vi "湿度显示前面板.vi"(0 "通道设置":u8=1 min=1 max=100, 1 "通讯设置":T1={"COM1", "Baud Rate"=19200, "Slave Address"=255}) -> (3 "光谱图像":cluster{dbl[], u16[]}(graph))   [LabVIEW 2018]
uses:
  <vilib>/Utility/file.llb/Read Delimited Spreadsheet (DBL).vi
  <vilib>/Utility/file.llb/Write To Spreadsheet File (DBL).vi
panel:
  in  "阈值":u16
  in  "连接":bool
  in  "选项卡控件":T2(tab)
  out "3通道":dbl[](array[numeric]) format="%#_7g"
  out "2通道":dbl[](array[numeric]) format="%#_7g"
  out "1通道":dbl[](array[numeric])=[1546.786, 1549.013] format="%#_7g"
  out "4通道":dbl[](array[numeric]) format="%#_7g"
  out "波形图表 20":dbl(graph)
  out "波形图表 19":dbl(graph)
  out "波形图表 18":dbl(graph)
  out "波形图表 17":dbl(graph)
  out "波形图表 16":dbl(graph)
  out "波形图表 15":dbl(graph)
  out "波形图表 14":dbl(graph)
  out "波形图表 13":dbl(graph)
  out "波形图表 12":dbl(graph)
  out "波形图表 11":dbl(graph)
  out "波形图表 10":dbl(graph)
  out "波形图表 9":dbl(graph)
  out "波形图表 8":dbl(graph)
  out "波形图表 7":dbl(graph)
  out "波形图表 6":dbl(graph)
  out "波形图表 5":dbl(graph)
  out "湿度1":dbl
  out "温度1":dbl
  out "湿度2":dbl
  out "温度2":dbl
  out "湿度3":dbl
  out "温度3":dbl
  out "湿度4":dbl
  out "温度4":dbl
  out "湿度5":dbl
  out "温度5":dbl
  out "湿度6":dbl
  out "温度6":dbl
  out "湿度7":dbl
  out "温度7":dbl
  out "湿度8":dbl
  out "温度8":dbl
  out "湿度9":dbl
  out "温度9":dbl
  out "湿度10":dbl
  out "温度10":dbl
  out "波形图表 2":dbl(graph)
  out "波形图表 3":dbl(graph)
  out "波形图表 4":dbl(graph)
  out "波形图表":dbl(graph)
  out "波形图表 40":dbl(graph)
  out "波形图表 39":dbl(graph)
  out "波形图表 38":dbl(graph)
  out "波形图表 37":dbl(graph)
  out "波形图表 36":dbl(graph)
  out "波形图表 35":dbl(graph)
  out "波形图表 34":dbl(graph)
  out "波形图表 33":dbl(graph)
  out "波形图表 32":dbl(graph)
  out "波形图表 31":dbl(graph)
  out "波形图表 30":dbl(graph)
  out "波形图表 29":dbl(graph)
  out "波形图表 28":dbl(graph)
  out "波形图表 27":dbl(graph)
  out "波形图表 26":dbl(graph)
  out "波形图表 25":dbl(graph)
  out "波形图表 24":dbl(graph)
  out "波形图表 23":dbl(graph)
  out "波形图表 22":dbl(graph)
  out "波形图表 21":dbl(graph)
  out "湿度5 2":dbl
  out "温度5 2":dbl
  out "湿度6 2":dbl
  out "温度6 2":dbl
  out "湿度7 2":dbl
  out "温度7 2":dbl
  out "湿度8 2":dbl
  out "温度8 2":dbl
  out "湿度9 2":dbl
  out "温度9 2":dbl
  out "湿度10 2":dbl
  out "温度10 2":dbl
  out "湿度1 2":dbl
  out "温度1 2":dbl
  out "湿度2 2":dbl
  out "温度2 2":dbl
  out "湿度3 2":dbl
  out "温度3 2":dbl
  out "湿度4 2":dbl
  out "温度4 2":dbl
  out "波形图表 60":dbl(graph)
  out "波形图表 59":dbl(graph)
  out "波形图表 58":dbl(graph)
  out "波形图表 57":dbl(graph)
  out "波形图表 56":dbl(graph)
  out "波形图表 55":dbl(graph)
  out "波形图表 54":dbl(graph)
  out "波形图表 53":dbl(graph)
  out "波形图表 52":dbl(graph)
  out "波形图表 51":dbl(graph)
  out "波形图表 50":dbl(graph)
  out "波形图表 49":dbl(graph)
  out "波形图表 48":dbl(graph)
  out "波形图表 47":dbl(graph)
  out "波形图表 46":dbl(graph)
  out "波形图表 45":dbl(graph)
  out "波形图表 44":dbl(graph)
  out "波形图表 43":dbl(graph)
  out "波形图表 42":dbl(graph)
  out "波形图表 41":dbl(graph)
  out "温度1 3":dbl
  out "湿度1 3":dbl
  out "温度4 3":dbl
  out "湿度4 3":dbl
  out "温度3 3":dbl
  out "湿度3 3":dbl
  out "温度2 3":dbl
  out "湿度2 3":dbl
  out "湿度5 3":dbl
  out "温度5 3":dbl
  out "湿度6 3":dbl
  out "温度6 3":dbl
  out "湿度7 3":dbl
  out "温度7 3":dbl
  out "湿度8 3":dbl
  out "温度8 3":dbl
  out "湿度9 3":dbl
  out "温度9 3":dbl
  out "湿度10 3":dbl
  out "温度10 3":dbl
  out "波形图表 80":dbl(graph)
  out "波形图表 79":dbl(graph)
  out "波形图表 78":dbl(graph)
  out "波形图表 77":dbl(graph)
  out "波形图表 76":dbl(graph)
  out "波形图表 75":dbl(graph)
  out "波形图表 74":dbl(graph)
  out "波形图表 73":dbl(graph)
  out "波形图表 72":dbl(graph)
  out "波形图表 71":dbl(graph)
  out "波形图表 70":dbl(graph)
  out "波形图表 69":dbl(graph)
  out "波形图表 68":dbl(graph)
  out "波形图表 67":dbl(graph)
  out "波形图表 66":dbl(graph)
  out "波形图表 65":dbl(graph)
  out "波形图表 64":dbl(graph)
  out "波形图表 63":dbl(graph)
  out "波形图表 62":dbl(graph)
  out "波形图表 61":dbl(graph)
  out "温度1 4":dbl
  out "湿度1 4":dbl
  out "湿度2 4":dbl
  out "温度2 4":dbl
  out "湿度3 4":dbl
  out "温度3 4":dbl
  out "湿度4 4":dbl
  out "温度4 4":dbl
  out "湿度5 4":dbl
  out "温度5 4":dbl
  out "湿度6 4":dbl
  out "温度6 4":dbl
  out "湿度7 4":dbl
  out "温度7 4":dbl
  out "湿度8 4":dbl
  out "温度8 4":dbl
  out "湿度9 4":dbl
  out "温度9 4":dbl
  out "湿度10 4":dbl
  out "温度10 4":dbl
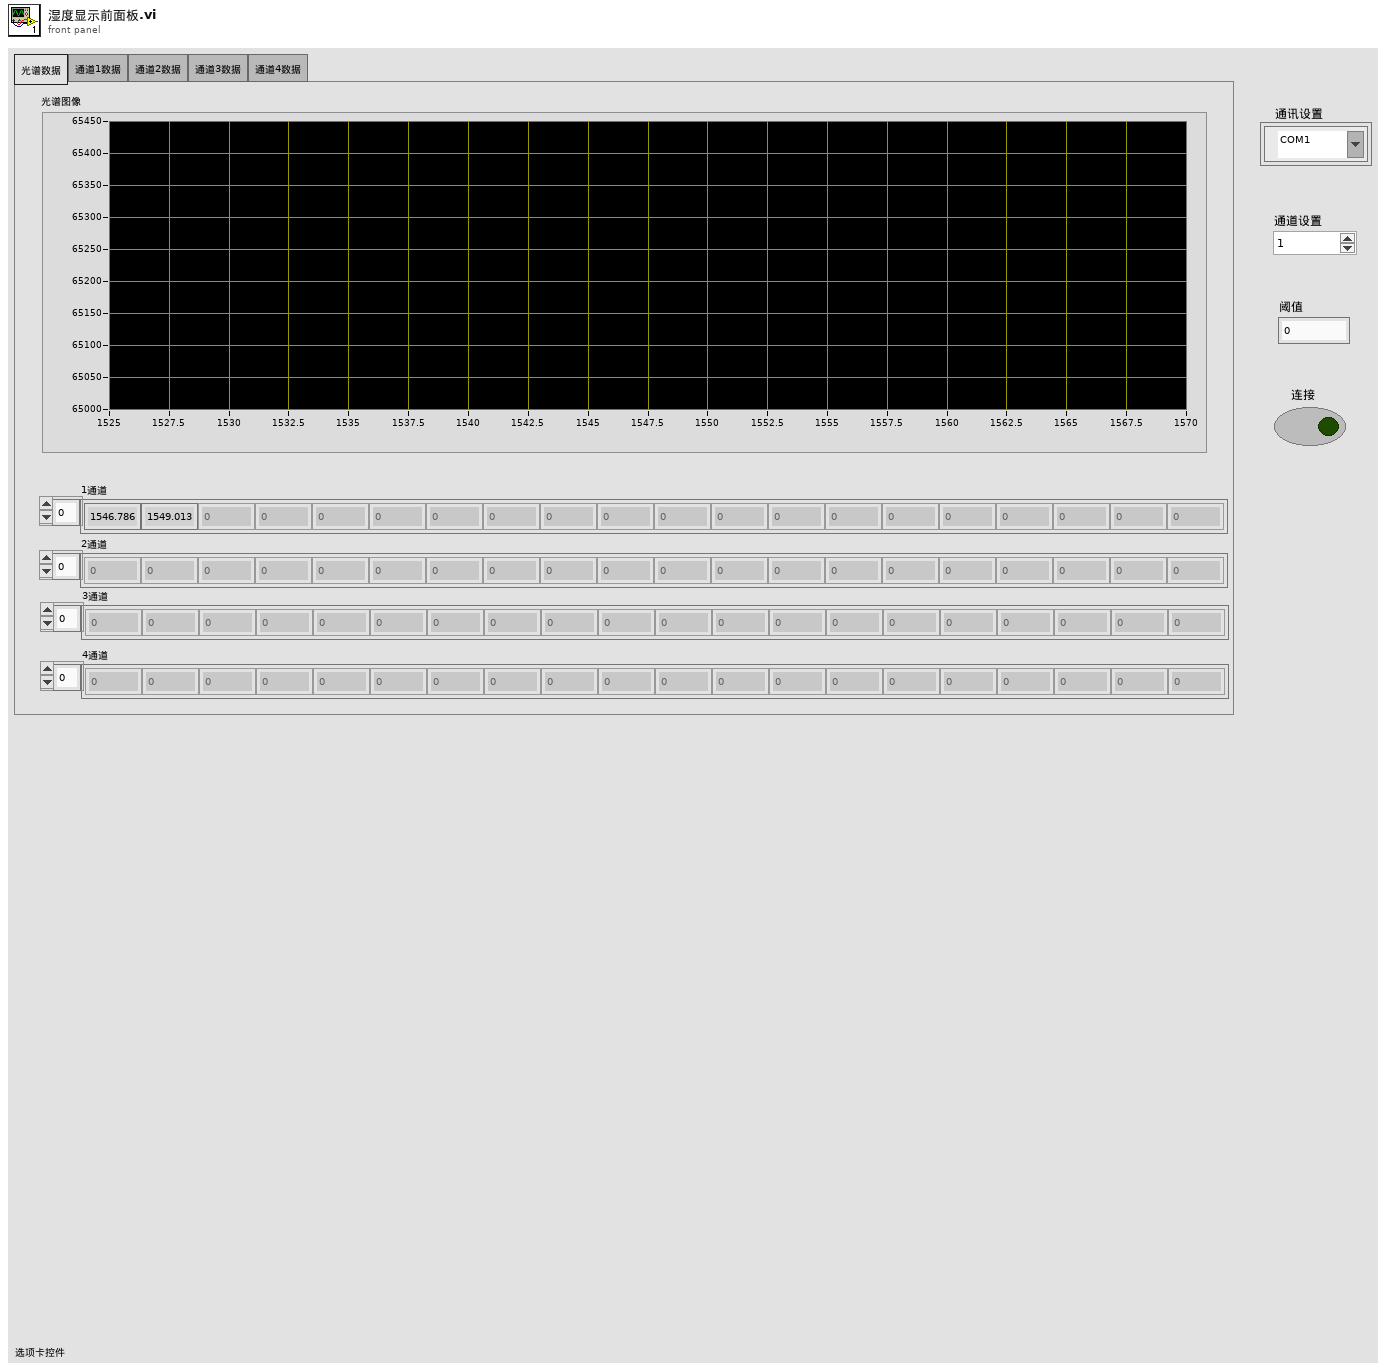
[diagram p1: front panel]
types:
  T1 = cluster{refnum<visa-resource-name>, "Baud Rate":u32, "Slave Address":u8}
  T2 = enum32{"光谱数据", "通道1数据", "通道2数据", "通道3数据", "通道4数据"}
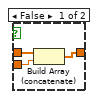
[diagram p2: hidden frame]
diagram:
  n1 = Unbundle By Name("通讯设置") -> ("Slave Address"=w5:u8)
  n2 = while {
    tunnel: w5 -> [w674]
    tunnel: "通讯设置" -> [w673]
    tunnel: [w672] -> w2
    tunnel: [w671] -> w1
    stop <- "连接" continue-if-true
    w678 = path "E:/湿度/四通道湿度结果" ("基路径")
    n3 = call "U8toHEX.vi"("data"=w674) -> ("HEX"=w726:string)  [unwired: 10 in]
    n4 = Concatenate Strings(w726, "B" ("write buffer")) -> (w736:string)
    n5 = call "CRC16.vi"("DATA"=w736) -> ("CRC-16"=w729:string)  [unwired: 1 in, 1 out]
    n6 = Concatenate Strings(w736, w729) -> (w732:string)
    n7 = call "Initialize.vi"("通讯设置 in"=w673) -> ("error out"=w734:errorcluster, "VISA resource name out"=w733:refnum<visa-resource-name>)  [unwired: 1 in, 3 out]
    n8 = VISA Write(VISA resource name=w733, write buffer=w732, error in (no error)=w734) -> (VISA resource name out=w730:refnum<visa-resource-name>, error out=w731:errorcluster)  [unwired: 1 out]
    n9 = flat-sequence {
      tunnel: w731 -> [w1062]
      tunnel: w730 -> [w1063]
      tunnel: [w1063] -> w744
      tunnel: [w1062] -> w743
      tunnel: [w1069] -> w728
      tunnel: [w1068] -> w727
      tunnel: [w1067] -> w725
      tunnel: w744 -> [w1066]
      tunnel: w743 -> [w1070]
      frame #0 {
        n10 = Wait (ms)(milliseconds to wait=u32 1000) -> ()  [unwired: 1 out]
      }
      frame #1 {
        n11 = property class="Instr" props=["Bytes at Port"](reference=w1066) -> (reference out=w1065:refnum<visa-resource-name>)  [unwired: 1 in, 2 out]
        n12 = VISA Read(VISA resource name=w1065, byte count=u32 8 ("Serial Settings:Number of Bytes at Serial Port"), error in (no error)=w1070) -> (VISA resource name out=w1069:refnum<visa-resource-name>, read buffer=w1068:string, error out=w1067:errorcluster)  [unwired: 1 out]
      }
    }
    n13 = flat-sequence {
      tunnel: [w751] -> w742
      tunnel: w728 -> [w751]
      tunnel: w725 -> [w750]
      tunnel: [w750] -> w741
      tunnel: [w749] -> w740
      tunnel: w727 -> [w749]
      tunnel: [w748] -> w739
      tunnel: w674 -> [w748]
      tunnel: [w747] -> w738
      tunnel: w726 -> [w747]
      tunnel: [w746] -> w737
      tunnel: "通道设置" -> [w746]
      tunnel: w742 -> [w789]
      tunnel: w741 -> [w788]
      tunnel: w740 -> [w787]
      tunnel: w739 -> [w776]
      tunnel: w738 -> [w765]
      tunnel: w737 -> [w781]
      tunnel: [w771] -> w503
      tunnel: [w770] -> w513
      tunnel: [w769] -> w505
      tunnel: [w763] -> w676
      tunnel: [w761] -> w675
      tunnel: [w752] -> w497
      tunnel: [w1060] -> w672
      tunnel: [w1059] -> w671
      tunnel: w676 -> [w1060]
      tunnel: w675 -> [w1059]
      frame #0 {
        n14 = Wait (ms)(milliseconds to wait=u32 1000) -> ()  [unwired: 1 out]
      }
      frame #1 {
        n15 = Decrement(x=w781) -> (x-1=w803:u8)
        n16 = String To Byte Array(string=w787) -> (unsigned byte array=w793:u8[])
        n17 = Concatenate Strings(w765, "C" ("write buffer")) -> (w780:string)
        n18 = call "U8toHEX.vi"("data"=w803) -> ("HEX"=w779:string)  [unwired: 10 in]
        n19 = Array Size(array=w793) -> (size(s)=w795:i32)
        n20 = call "set test state（三态）.vi"("error in"=w788, "Slave Address"=w776, "启动单次"=TRUE, "VISA resource name in"=w789) -> ("error out"=w801:errorcluster, "VISA resource name out"=w797:refnum<visa-resource-name>)  [unwired: 2 in, 2 out]
        n21 = Concatenate Strings(w780, w779) -> (w778:string)
        n22 = Divide(x=w795, y=2 ("offset (0)")) -> (x/y=w796:dbl)
        n23 = for {
          N: w796 -> [_]
          tunnel: w793 -> [w1056]
          tunnel: [w1049] -> w792 mode=indexing
          i -> [w1057]
          n24 = Multiply(x=w1057, y=2) -> (x*y=w1054:i32)
          n25 = Array Subset(array=w1056, index=w1054, length=2) -> (w1048:u8[])
          n26 = Index Array(array=w1048) -> (element #1=w1053:u8, element #2=w1050:u8)  [unwired: 2 in]
          n27 = Multiply(x=w1053, y=u16 256) -> (x*y=w1051:u16)
          n28 = Add(x=w1051, y=w1050) -> (x+y=w1049:u16)
        }
        n29 = call "CRC16.vi"("DATA"=w778) -> ("CRC-16"=w800:string)  [unwired: 1 in, 1 out]
        n30 = Concatenate Strings(w778, w800) -> (w799:string)
        n31 = VISA Write(VISA resource name=w797, write buffer=w799, error in (no error)=w801) -> (VISA resource name out=w802:refnum<visa-resource-name>, error out=w798:errorcluster)  [unwired: 1 out]
        n32 = Index Array(array=w792) -> (element #1=w791:u16, element #2=w790:u16, element #3=w766:u16)  [unwired: 3 in]
        n33 = flat-sequence {
          tunnel: w791 -> [w824]
          tunnel: w790 -> [w823]
          tunnel: w802 -> [w821]
          tunnel: w798 -> [w819]
          tunnel: w766 -> [w807]
          tunnel: [w826] -> w785
          tunnel: [w825] -> w784
          tunnel: [w815] -> w783
          tunnel: [w814] -> w782
          tunnel: [w804] -> w754
          tunnel: w765 -> [w874]
          tunnel: w776 -> [w869]
          tunnel: w782 -> [w873]
          tunnel: w783 -> [w872]
          tunnel: w784 -> [w904]
          tunnel: w785 -> [_]
          tunnel: [w871] -> w768
          tunnel: [w870] -> w767
          tunnel: [w868] -> w764
          tunnel: w754 -> [w867]
          tunnel: [w867] -> w753
          tunnel: w768 -> [w930]
          tunnel: w767 -> [w931]
          tunnel: w765 -> [w936]
          tunnel: w764 -> [w935]
          tunnel: [w934] -> w762
          tunnel: [w933] -> w760
          tunnel: [w932] -> w759
          tunnel: w753 -> [w929]
          tunnel: [w1047] -> w763
          tunnel: w762 -> [w1047]
          tunnel: [w1046] -> w761
          tunnel: w760 -> [w1046]
          tunnel: [w1045] -> w758
          tunnel: w759 -> [w1045]
          tunnel: [w1045] -> w757
          tunnel: [w1045] -> w756
          tunnel: [w1045] -> w755
          frame #0 {
            n34 = Multiply(x=w807, y=u16 2) -> (x*y=w804:u16)
            n35 = Divide(x=w824, y=u16 1000) -> (x/y=w829:dbl)
            n36 = Tick Count (ms)() -> (millisecond timer value=w816:u32)
            n37 = while {
              tunnel: [""] -> w831
              tunnel: w821 -> [w857]
              tunnel: [w856] -> w820
              tunnel: w819 -> [w855]
              tunnel: [w853] -> w818
              tunnel: [w854] -> w817
              tunnel: w816 -> [w849]
              tunnel: w804 -> [w843]
              stop <- w844 stop-if-true
              n38 = Tick Count (ms)() -> (millisecond timer value=w850:u32)
              n39 = property class="Instr"(reference=w857, error in=w855) -> (reference out=w856:refnum<visa-resource-name>, error out=w853:errorcluster, "Bytes at Port"=w854:u32)
              n40 = Subtract(x=w850, y=w849) -> (x-y=w848:u32)
              n41 = Unbundle By Name(w853) -> ("status"=w852:bool)
              n42 = Equal?(x=w843, y=w854) -> (x = y?=w851:bool)
              n43 = Greater Or Equal?(x=w848, y=u32 5000) -> (x >= y?=w846:bool)
              n44 = Or(x=w851, y=w852) -> (x .or. y?=w845:bool)
              n45 = Or(x=w846, y=w845) -> (x .or. y?=w844:bool)
            }
            n46 = Add(x=w829, y=1520.0) -> (x+y=w827:dbl)
            n47 = VISA Read(VISA resource name=w820, byte count=w817, error in (no error)=w818) -> (VISA resource name out=w815:refnum<visa-resource-name>, read buffer=w822:string, error out=w814:errorcluster)  [unwired: 1 out]
            n48 = Concatenate Strings(w831, w822) -> (w805:string)
            n49 = String To Byte Array(string=w805) -> (unsigned byte array=w811:u8[])
            n50 = Array Size(array=w811) -> (size(s)=w810:i32)
            n51 = Divide(x=w810, y=2 ("offset (0)")) -> (x/y=w809:dbl)
            n52 = for {
              N: w809 -> [_]
              tunnel: w811 -> [w840]
              tunnel: [w833] -> w808 mode=indexing
              i -> [w841]
              n53 = Multiply(x=w841, y=2) -> (x*y=w838:i32)
              n54 = Array Subset(array=w840, index=w838, length=2) -> (w832:u8[])
              n55 = Index Array(array=w832) -> (element #1=w837:u8, element #2=w834:u8)  [unwired: 2 in]
              n56 = Multiply(x=w837, y=u16 256) -> (x*y=w835:u16)
              n57 = Add(x=w835, y=w834) -> (x+y=w833:u16)
            }
            n58 = for {
              N: w807 -> [_]
              tunnel: w827 -> [w861]
              tunnel: w823 -> [w864]
              tunnel: [w859] -> w813 mode=indexing
              i -> [w865]
              n59 = Multiply(x=w864, y=w865) -> (x*y=w863:i32)
              n60 = Divide(x=w863, y=1000) -> (x/y=w860:dbl)
              n61 = Add(x=w861, y=w860) -> (x+y=w859:dbl)
            }
            n62 = Bundle(w813, w808) -> (w825:cluster{dbl[], u16[]})  [unwired: 1 in]
            n63 = Build Array(w813, w808) -> (w826:dbl[][])
          }
          frame #1 {
            n64 = Wait (ms)(milliseconds to wait=u32 1000) -> ()  [unwired: 1 out]
            n65 = call "set test state（三态）.vi"("error in"=w873, "Slave Address"=w869, "启动单次"=TRUE, "VISA resource name in"=w872) -> ("error out"=w893:errorcluster, "VISA resource name out"=w892:refnum<visa-resource-name>)  [unwired: 2 in, 2 out]
            n66 = Concatenate Strings(w874, "\u0004" ("write buffer")) -> (w886:string)
            n67 = call "U8toHEX.vi"("data"=u8 1) -> ("HEX"=w878:string)  [unwired: 10 in]
            n68 = Concatenate Strings(w886, w878) -> (w885:string)
            n69 = call "U8toHEX.vi"("data"=u8 194) -> ("HEX"=w876:string)  [unwired: 10 in]
            n70 = Concatenate Strings(w885, w876) -> (w884:string)
            n71 = call "U8toHEX.vi"("data"=u8 0) -> ("HEX"=w882:string)  [unwired: 10 in]
            n72 = Concatenate Strings(w884, w882) -> (w883:string)
            n73 = call "U8toHEX.vi"("data"=u8 120) -> ("HEX"=w889:string)  [unwired: 10 in]
            n74 = Concatenate Strings(w883, w889) -> (w887:string)
            n75 = call "CRC16.vi"("DATA"=w887) -> ("CRC-16"=w880:string)  [unwired: 1 in, 1 out]
            n76 = Concatenate Strings(w887, w880) -> (w879:string)
            n77 = VISA Write(VISA resource name=w892, write buffer=w879, error in (no error)=w893) -> (VISA resource name out=w896:refnum<visa-resource-name>, error out=w897:errorcluster)  [unwired: 1 out]
            n78 = Tick Count (ms)() -> (millisecond timer value=w898:u32)
            n79 = while {
              tunnel: [""] -> w903
              tunnel: w896 -> [w926]
              tunnel: [w925] -> w901
              tunnel: w897 -> [w924]
              tunnel: [w922] -> w900
              tunnel: [w923] -> w899
              tunnel: w898 -> [w918]
              tunnel: w867 -> [w912]
              stop <- w913 stop-if-true
              n80 = Tick Count (ms)() -> (millisecond timer value=w919:u32)
              n81 = property class="Instr"(reference=w926, error in=w924) -> (reference out=w925:refnum<visa-resource-name>, error out=w922:errorcluster, "Bytes at Port"=w923:u32)
              n82 = Subtract(x=w919, y=w918) -> (x-y=w917:u32)
              n83 = Unbundle By Name(w922) -> ("status"=w921:bool)
              n84 = Equal?(x=w912, y=w923) -> (x = y?=w920:bool)
              n85 = Greater Or Equal?(x=w917, y=u32 2000) -> (x >= y?=w915:bool)
              n86 = Or(x=w920, y=w921) -> (x .or. y?=w914:bool)
              n87 = Or(x=w915, y=w914) -> (x .or. y?=w913:bool)
            }
            n88 = VISA Read(VISA resource name=w901, byte count=w899, error in (no error)=w900) -> (VISA resource name out=w870:refnum<visa-resource-name>, read buffer=w902:string, error out=w871:errorcluster)  [unwired: 1 out]
            n89 = Concatenate Strings(w903, w902) -> (w894:string)
            n90 = for {
              N: 4 -> [_]
              tunnel: w894 -> [w911]
              tunnel: [w910] -> w868 mode=indexing
              i -> [w909]
              w905 = 60 ("x")
              n91 = Multiply(x=w905, y=w909) -> (x*y=w908:i32)
              n92 = Add(x=w908, y=3) -> (x+y=w906:i32)
              n93 = String Subset(string=w911, offset (0)=w906, length (rest)=w905) -> (substring=w910:string)
            }
            "光谱图像" <- w904
          }
          frame #2 {
            w938 = 4
            (unwired) 4
            n94 = Concatenate Strings(w936, "\u0004" ("write buffer")) -> (w951:string)
            n95 = Wait (ms)(milliseconds to wait=u32 1000) -> ()  [unwired: 1 out]
            n96 = call "U8toHEX.vi"("data"=u8 0) -> ("HEX"=w943:string)  [unwired: 10 in]
            n97 = Concatenate Strings(w951, w943) -> (w950:string)
            n98 = call "U8toHEX.vi"("data"=u8 200) -> ("HEX"=w941:string)  [unwired: 10 in]
            n99 = Concatenate Strings(w950, w941) -> (w949:string)
            n100 = call "U8toHEX.vi"("data"=u8 0) -> ("HEX"=w947:string)  [unwired: 10 in]
            n101 = Concatenate Strings(w949, w947) -> (w948:string)
            n102 = call "U8toHEX.vi"("data"=u8 120) -> ("HEX"=w954:string)  [unwired: 10 in]
            n103 = Concatenate Strings(w948, w954) -> (w952:string)
            n104 = call "CRC16.vi"("DATA"=w952) -> ("CRC-16"=w945:string)  [unwired: 1 in, 1 out]
            n105 = Concatenate Strings(w952, w945) -> (w944:string)
            n106 = VISA Write(VISA resource name=w931, write buffer=w944, error in (no error)=w930) -> (VISA resource name out=w956:refnum<visa-resource-name>, error out=w957:errorcluster)  [unwired: 1 out]
            n107 = Tick Count (ms)() -> (millisecond timer value=w958:u32)
            n108 = while {
              tunnel: [""] -> w963
              tunnel: w956 -> [w1042]
              tunnel: [w1041] -> w961
              tunnel: w957 -> [w1040]
              tunnel: [w1038] -> w960
              tunnel: [w1039] -> w959
              tunnel: w958 -> [w1034]
              tunnel: w929 -> [w1028]
              stop <- w1029 stop-if-true
              n109 = Tick Count (ms)() -> (millisecond timer value=w1035:u32)
              n110 = property class="Instr"(reference=w1042, error in=w1040) -> (reference out=w1041:refnum<visa-resource-name>, error out=w1038:errorcluster, "Bytes at Port"=w1039:u32)
              n111 = Subtract(x=w1035, y=w1034) -> (x-y=w1033:u32)
              n112 = Unbundle By Name(w1038) -> ("status"=w1037:bool)
              n113 = Equal?(x=w1028, y=w1039) -> (x = y?=w1036:bool)
              n114 = Greater Or Equal?(x=w1033, y=u32 2000) -> (x >= y?=w1031:bool)
              n115 = Or(x=w1036, y=w1037) -> (x .or. y?=w1030:bool)
              n116 = Or(x=w1031, y=w1030) -> (x .or. y?=w1029:bool)
            }
            n117 = VISA Read(VISA resource name=w961, byte count=w959, error in (no error)=w960) -> (VISA resource name out=w934:refnum<visa-resource-name>, read buffer=w962:string, error out=w933:errorcluster)  [unwired: 1 out]
            n118 = Concatenate Strings(w963, w962) -> (w939:string)
            n119 = for {
              N: w938 -> [_]
              tunnel: w939 -> [w970]
              tunnel: [w969] -> w937 mode=indexing
              i -> [w968]
              w964 = 60 ("x")
              n120 = Multiply(x=w964, y=w968) -> (x*y=w967:i32)
              n121 = Add(x=w967, y=3) -> (x+y=w965:i32)
              n122 = String Subset(string=w970, offset (0)=w965, length (rest)=w964) -> (substring=w969:string)
            }
            n123 = for {
              N: w938 -> [_]
              tunnel: w935 -> [w981]
              tunnel: w937 -> [w977]
              tunnel: [w971] -> w932 mode=indexing
              i -> [w978]
              w974 = 20
              n124 = Index Array(array=w981, index=w978) -> (element=w980:string)
              n125 = Index Array(array=w977, index=w978) -> (element=w979:string)
              n126 = String To Byte Array(string=w980) -> (unsigned byte array=w982:u8[])
              n127 = String To Byte Array(string=w979) -> (unsigned byte array=w976:u8[])
              n128 = for {
                N: w974 -> [_]
                tunnel: w982 -> [w1025]
                tunnel: w976 -> [w1009]
                tunnel: [w1004] -> w975 mode=indexing
                i -> [w1003]
                n129 = Multiply(x=w1003, y=2) -> (x*y=w1018:i32)
                n130 = Multiply(x=w1003, y=2) -> (x*y=w1010:i32)
                n131 = Array Subset(array=w1025, index=w1018, length=2) -> (w1019:u8[])
                n132 = Array Subset(array=w1009, index=w1010, length=2) -> (w1011:u8[])
                n133 = Index Array(array=w1019) -> (element #1=w1023:u8, element #2=w1020:u8)  [unwired: 2 in]
                n134 = Index Array(array=w1011) -> (element #1=w1015:u8, element #2=w1012:u8)  [unwired: 2 in]
                n135 = Multiply(x=w1023, y=u16 256) -> (x*y=w1021:u16)
                n136 = Multiply(x=w1015, y=u16 256) -> (x*y=w1013:u16)
                n137 = Add(x=w1021, y=w1020) -> (x+y=w1008:u16)
                n138 = Add(x=w1013, y=w1012) -> (x+y=w1005:u16)
                n139 = Greater Or Equal?(x=w1008, y="阈值") -> (x >= y?=w1006:bool)
                n140 = case shown="真" w1006 {
                  tunnel: w1005 -> [_ w1027]
                  tunnel: [_ w1027] -> w1004
                  frame False {
                  }
                  frame True {
                  }
                }
              }
              n141 = for {
                N: w974 -> [_]
                tunnel: w975 -> [w1001]
                tunnel: [w993] -> w972 mode=indexing
                i -> [w998]
                n142 = Index Array(array=w1001, index=w998) -> (element=w997:u16)
                n143 = Divide(x=w997, y=1000) -> (x/y=w999:dbl)
                n144 = Add(x=1520.0, y=w999) -> (x+y=w992:dbl)
                n145 = Greater?(x=w992, y=1520.0) -> (0:w994:bool)
                n146 = case shown="真" w994 {
                  tunnel: [_ w1002] -> w993
                  tunnel: w992 -> [_ w1002]
                  frame False {
                  }
                  frame True {
                  }
                }
              }
              n147 = for {
                tunnel: w972 -> [w985] mode=indexing
                shift-right: [w984] -> w971
                shift-left: dbl[] [] -> [w983]
                n148 = Equal?(x=w985, y=0.0) -> (x = y?=w986:bool)
                n149 = case shown="真" w986 {
                  tunnel: [w989 w991] -> w984
                  tunnel: w985 -> [w990 _]
                  tunnel: w983 -> [w988 w991]
                  frame False {
                    n150 = Build Array (concatenate)(w988, w990) -> (w989:dbl[])
                  }
                  frame True {
                  }
                }
              }
            }
          }
          frame #3 {
            n151 = Wait (ms)(milliseconds to wait=u32 1000) -> ()  [unwired: 1 out]
          }
        }
        n152 = Index Array(array=w757, index (row)=1 ("索引 (行)")) -> (element=w769:dbl[])  [unwired: 1 in]
        "2通道" <- w769
        n153 = Index Array(array=w758, index (row)=0 ("索引 (行)")) -> (element=w770:dbl[])  [unwired: 1 in]
        "1通道" <- w770
        n154 = Index Array(array=w755, index (row)=3 ("索引 (行)")) -> (element=w752:dbl[])  [unwired: 1 in]
        "4通道" <- w752
        n155 = Index Array(array=w756, index (row)=2 ("索引 (行)")) -> (element=w771:dbl[])  [unwired: 1 in]
        "3通道" <- w771
      }
      frame #2 {
      }
    }
    n156 = call-poly <vilib>:"Read Delimited Spreadsheet.vi"("file path (dialog if empty)"=path "E:/湿度/通道一标定文件.txt") -> ("all rows"=w145:dbl[][])  [unwired: 9 in, 5 out]
    n157 = call-poly <vilib>:"Read Delimited Spreadsheet.vi"("file path (dialog if empty)"=path "E:/湿度/通道二标定文件.txt") -> ("all rows"=w411:dbl[][])  [unwired: 9 in, 5 out]
    n158 = call-poly <vilib>:"Read Delimited Spreadsheet.vi"("file path (dialog if empty)"=path "E:/湿度/通道四标定文件.txt") -> ("all rows"=w309:dbl[][])  [unwired: 9 in, 5 out]
    n159 = call-poly <vilib>:"Read Delimited Spreadsheet.vi"("file path (dialog if empty)"=path "E:/湿度/通道三标定文件.txt") -> ("all rows"=w207:dbl[][])  [unwired: 9 in, 5 out]
    n160 = Index Array(array=w145, index (row)=0 ("索引 (行)")) -> (element=w144:dbl[])  [unwired: 1 in]
    n161 = Index Array(array=w145, index (row)=1 ("索引 (行)")) -> (element=w127:dbl[])  [unwired: 1 in]
    n162 = Index Array(array=w145, index (row)=2 ("索引 (行)")) -> (element=w126:dbl[])  [unwired: 1 in]
    n163 = Index Array(array=w145, index (row)=3 ("索引 (行)")) -> (element=w125:dbl[])  [unwired: 1 in]
    n164 = Index Array(array=w145, index (row)=4 ("索引 (行)")) -> (element=w110:dbl[])  [unwired: 1 in]
    n165 = Index Array(array=w145, index (row)=7 ("索引 (行)")) -> (element=w87:dbl[])  [unwired: 1 in]
    n166 = Index Array(array=w505, index=0 ("索引")) -> (element=w631:dbl)
    n167 = Index Array(array=w505, index=1 ("索引")) -> (element=w629:dbl)
    n168 = Index Array(array=w505, index=2 ("索引")) -> (element=w627:dbl)
    n169 = Index Array(array=w505, index=3 ("索引")) -> (element=w625:dbl)
    n170 = Index Array(array=w505, index=4 ("索引")) -> (element=w623:dbl)
    n171 = Index Array(array=w505, index=5 ("索引")) -> (element=w621:dbl)
    n172 = Index Array(array=w505, index=6 ("索引")) -> (element=w619:dbl)
    n173 = Index Array(array=w505, index=7 ("索引")) -> (element=w617:dbl)
    n174 = Index Array(array=w505, index=8 ("索引")) -> (element=w615:dbl)
    n175 = Index Array(array=w505, index=9 ("索引")) -> (element=w613:dbl)
    n176 = Index Array(array=w513, index=0 ("索引")) -> (element=w669:dbl)
    n177 = Index Array(array=w513, index=1 ("索引")) -> (element=w667:dbl)
    n178 = Index Array(array=w513, index=2 ("索引")) -> (element=w665:dbl)
    n179 = Index Array(array=w513, index=3 ("索引")) -> (element=w663:dbl)
    n180 = Index Array(array=w513, index=4 ("索引")) -> (element=w661:dbl)
    n181 = Index Array(array=w513, index=5 ("索引")) -> (element=w659:dbl)
    n182 = Index Array(array=w513, index=6 ("索引")) -> (element=w657:dbl)
    n183 = Index Array(array=w513, index=7 ("索引")) -> (element=w655:dbl)
    n184 = Index Array(array=w513, index=8 ("索引")) -> (element=w653:dbl)
    n185 = Index Array(array=w513, index=9 ("索引")) -> (element=w651:dbl)
    n186 = Index Array(array=w497, index=0 ("索引")) -> (element=w552:dbl)
    n187 = Index Array(array=w497, index=1 ("索引")) -> (element=w550:dbl)
    n188 = Index Array(array=w497, index=2 ("索引")) -> (element=w548:dbl)
    n189 = Index Array(array=w497, index=3 ("索引")) -> (element=w546:dbl)
    n190 = Index Array(array=w497, index=4 ("索引")) -> (element=w544:dbl)
    n191 = Index Array(array=w497, index=5 ("索引")) -> (element=w542:dbl)
    n192 = Index Array(array=w497, index=6 ("索引")) -> (element=w540:dbl)
    n193 = Index Array(array=w497, index=7 ("索引")) -> (element=w538:dbl)
    n194 = Index Array(array=w497, index=8 ("索引")) -> (element=w536:dbl)
    n195 = Index Array(array=w497, index=9 ("索引")) -> (element=w534:dbl)
    n196 = Index Array(array=w503, index=0 ("索引")) -> (element=w591:dbl)
    n197 = Index Array(array=w503, index=1 ("索引")) -> (element=w589:dbl)
    n198 = Index Array(array=w503, index=2 ("索引")) -> (element=w587:dbl)
    n199 = Index Array(array=w503, index=3 ("索引")) -> (element=w585:dbl)
    n200 = Index Array(array=w503, index=4 ("索引")) -> (element=w583:dbl)
    n201 = Index Array(array=w503, index=5 ("索引")) -> (element=w581:dbl)
    n202 = Index Array(array=w503, index=6 ("索引")) -> (element=w579:dbl)
    n203 = Index Array(array=w503, index=7 ("索引")) -> (element=w577:dbl)
    n204 = Index Array(array=w503, index=8 ("索引")) -> (element=w575:dbl)
    n205 = Index Array(array=w503, index=9 ("索引")) -> (element=w573:dbl)
    n206 = Index Array(array=w411, index (row)=0 ("索引 (行)")) -> (element=w410:dbl[])  [unwired: 1 in]
    n207 = Index Array(array=w411, index (row)=1 ("索引 (行)")) -> (element=w393:dbl[])  [unwired: 1 in]
    n208 = Index Array(array=w411, index (row)=2 ("索引 (行)")) -> (element=w392:dbl[])  [unwired: 1 in]
    n209 = Index Array(array=w411, index (row)=3 ("索引 (行)")) -> (element=w391:dbl[])  [unwired: 1 in]
    n210 = Index Array(array=w411, index (row)=4 ("索引 (行)")) -> (element=w376:dbl[])  [unwired: 1 in]
    n211 = Index Array(array=w411, index (row)=5 ("索引 (行)")) -> (element=w355:dbl[])  [unwired: 1 in]
    n212 = Index Array(array=w411, index (row)=6 ("索引 (行)")) -> (element=w354:dbl[])  [unwired: 1 in]
    n213 = Index Array(array=w411, index (row)=7 ("索引 (行)")) -> (element=w353:dbl[])  [unwired: 1 in]
    n214 = Index Array(array=w411, index (row)=8 ("索引 (行)")) -> (element=w352:dbl[])  [unwired: 1 in]
    n215 = Index Array(array=w411, index (row)=9 ("索引 (行)")) -> (element=w351:dbl[])  [unwired: 1 in]
    n216 = Index Array(array=w144, index=1 ("索引")) -> (element=w23:dbl)
    n217 = Index Array(array=w144, index=0 ("索引")) -> (element=w24:dbl)
    n218 = Index Array(array=w144, index=2 ("索引")) -> (element=w44:dbl)
    n219 = Index Array(array=w144, index=3 ("索引")) -> (element=w43:dbl)
    n220 = Index Array(array=w127, index=1 ("索引")) -> (element=w21:dbl)
    n221 = Index Array(array=w127, index=0 ("索引")) -> (element=w22:dbl)
    n222 = Index Array(array=w127, index=2 ("索引")) -> (element=w42:dbl)
    n223 = Index Array(array=w127, index=3 ("索引")) -> (element=w41:dbl)
    n224 = Index Array(array=w126, index=1 ("索引")) -> (element=w19:dbl)
    n225 = Index Array(array=w126, index=0 ("索引")) -> (element=w20:dbl)
    n226 = Index Array(array=w126, index=2 ("索引")) -> (element=w40:dbl)
    n227 = Index Array(array=w126, index=3 ("索引")) -> (element=w39:dbl)
    n228 = Index Array(array=w125, index=1 ("索引")) -> (element=w17:dbl)
    n229 = Index Array(array=w125, index=0 ("索引")) -> (element=w18:dbl)
    n230 = Index Array(array=w125, index=2 ("索引")) -> (element=w38:dbl)
    n231 = Index Array(array=w125, index=3 ("索引")) -> (element=w37:dbl)
    n232 = Index Array(array=w110, index=1 ("索引")) -> (element=w15:dbl)
    n233 = Index Array(array=w110, index=0 ("索引")) -> (element=w16:dbl)
    n234 = Index Array(array=w110, index=2 ("索引")) -> (element=w36:dbl)
    n235 = Index Array(array=w110, index=3 ("索引")) -> (element=w35:dbl)
    n236 = Index Array(array=w145, index (row)=5 ("索引 (行)")) -> (element=w89:dbl[])  [unwired: 1 in]
    n237 = Index Array(array=w145, index (row)=6 ("索引 (行)")) -> (element=w88:dbl[])  [unwired: 1 in]
    n238 = Index Array(array=w145, index (row)=8 ("索引 (行)")) -> (element=w86:dbl[])  [unwired: 1 in]
    n239 = Index Array(array=w145, index (row)=9 ("索引 (行)")) -> (element=w85:dbl[])  [unwired: 1 in]
    n240 = Index Array(array=w87, index=1 ("索引")) -> ()  [unwired: 1 out]
    n241 = Index Array(array=w309, index (row)=0 ("索引 (行)")) -> (element=w308:dbl[])  [unwired: 1 in]
    n242 = Index Array(array=w309, index (row)=1 ("索引 (行)")) -> (element=w291:dbl[])  [unwired: 1 in]
    n243 = Index Array(array=w309, index (row)=2 ("索引 (行)")) -> (element=w290:dbl[])  [unwired: 1 in]
    n244 = Index Array(array=w309, index (row)=3 ("索引 (行)")) -> (element=w289:dbl[])  [unwired: 1 in]
    n245 = Index Array(array=w309, index (row)=4 ("索引 (行)")) -> (element=w274:dbl[])  [unwired: 1 in]
    n246 = Index Array(array=w309, index (row)=5 ("索引 (行)")) -> (element=w253:dbl[])  [unwired: 1 in]
    n247 = Index Array(array=w309, index (row)=6 ("索引 (行)")) -> (element=w252:dbl[])  [unwired: 1 in]
    n248 = Index Array(array=w309, index (row)=7 ("索引 (行)")) -> (element=w251:dbl[])  [unwired: 1 in]
    n249 = Index Array(array=w309, index (row)=8 ("索引 (行)")) -> (element=w250:dbl[])  [unwired: 1 in]
    n250 = Index Array(array=w309, index (row)=9 ("索引 (行)")) -> (element=w249:dbl[])  [unwired: 1 in]
    n251 = Index Array(array=w207, index (row)=0 ("索引 (行)")) -> (element=w206:dbl[])  [unwired: 1 in]
    n252 = Index Array(array=w207, index (row)=1 ("索引 (行)")) -> (element=w189:dbl[])  [unwired: 1 in]
    n253 = Index Array(array=w207, index (row)=2 ("索引 (行)")) -> (element=w188:dbl[])  [unwired: 1 in]
    n254 = Index Array(array=w207, index (row)=3 ("索引 (行)")) -> (element=w187:dbl[])  [unwired: 1 in]
    n255 = Index Array(array=w207, index (row)=4 ("索引 (行)")) -> (element=w172:dbl[])  [unwired: 1 in]
    n256 = Index Array(array=w207, index (row)=5 ("索引 (行)")) -> (element=w151:dbl[])  [unwired: 1 in]
    n257 = Index Array(array=w207, index (row)=6 ("索引 (行)")) -> (element=w150:dbl[])  [unwired: 1 in]
    n258 = Index Array(array=w207, index (row)=7 ("索引 (行)")) -> (element=w149:dbl[])  [unwired: 1 in]
    n259 = Index Array(array=w207, index (row)=8 ("索引 (行)")) -> (element=w148:dbl[])  [unwired: 1 in]
    n260 = Index Array(array=w207, index (row)=9 ("索引 (行)")) -> (element=w147:dbl[])  [unwired: 1 in]
    n261 = Index Array(array=w505, index=10 ("索引")) -> (element=w611:dbl)
    n262 = Index Array(array=w505, index=11 ("索引")) -> (element=w609:dbl)
    n263 = Index Array(array=w505, index=12 ("索引")) -> (element=w607:dbl)
    n264 = Index Array(array=w505, index=13 ("索引")) -> (element=w605:dbl)
    n265 = Index Array(array=w505, index=14 ("索引")) -> (element=w603:dbl)
    n266 = Index Array(array=w505, index=15 ("索引")) -> (element=w601:dbl)
    n267 = Index Array(array=w505, index=16 ("索引")) -> (element=w599:dbl)
    n268 = Index Array(array=w505, index=17 ("索引")) -> (element=w597:dbl)
    n269 = Index Array(array=w505, index=18 ("索引")) -> (element=w595:dbl)
    n270 = Index Array(array=w505, index=19 ("索引")) -> (element=w593:dbl)
    n271 = Index Array(array=w513, index=10 ("索引")) -> (element=w649:dbl)
    n272 = Index Array(array=w513, index=13 ("索引")) -> (element=w645:dbl)
    n273 = Index Array(array=w513, index=14 ("索引")) -> (element=w643:dbl)
    n274 = Index Array(array=w513, index=15 ("索引")) -> (element=w641:dbl)
    n275 = Index Array(array=w513, index=16 ("索引")) -> (element=w639:dbl)
    n276 = Index Array(array=w513, index=17 ("索引")) -> (element=w637:dbl)
    n277 = Index Array(array=w513, index=18 ("索引")) -> (element=w635:dbl)
    n278 = Index Array(array=w513, index=19 ("索引")) -> (element=w633:dbl)
    n279 = Index Array(array=w513, index=11 ("索引")) -> (element=w230:dbl)
    n280 = Index Array(array=w513, index=12 ("索引")) -> (element=w229:dbl)
    n281 = Index Array(array=w497, index=10 ("索引")) -> (element=w532:dbl)
    n282 = Index Array(array=w497, index=11 ("索引")) -> (element=w530:dbl)
    n283 = Index Array(array=w497, index=12 ("索引")) -> (element=w528:dbl)
    n284 = Index Array(array=w497, index=13 ("索引")) -> (element=w526:dbl)
    n285 = Index Array(array=w497, index=14 ("索引")) -> (element=w524:dbl)
    n286 = Index Array(array=w497, index=15 ("索引")) -> (element=w522:dbl)
    n287 = Index Array(array=w497, index=16 ("索引")) -> (element=w520:dbl)
    n288 = Index Array(array=w497, index=17 ("索引")) -> (element=w518:dbl)
    n289 = Index Array(array=w497, index=18 ("索引")) -> (element=w516:dbl)
    n290 = Index Array(array=w497, index=19 ("索引")) -> (element=w514:dbl)
    n291 = Index Array(array=w503, index=10 ("索引")) -> (element=w474:dbl)
    n292 = Index Array(array=w503, index=11 ("索引")) -> (element=w570:dbl)
    n293 = Index Array(array=w503, index=12 ("索引")) -> (element=w568:dbl)
    n294 = Index Array(array=w503, index=13 ("索引")) -> (element=w566:dbl)
    n295 = Index Array(array=w503, index=14 ("索引")) -> (element=w564:dbl)
    n296 = Index Array(array=w503, index=15 ("索引")) -> (element=w562:dbl)
    n297 = Index Array(array=w503, index=16 ("索引")) -> (element=w560:dbl)
    n298 = Index Array(array=w503, index=17 ("索引")) -> (element=w558:dbl)
    n299 = Index Array(array=w503, index=18 ("索引")) -> (element=w556:dbl)
    n300 = Index Array(array=w503, index=19 ("索引")) -> (element=w554:dbl)
    n301 = formula code="y=(x-a)/b;"("x"=w669, "a"=w23, "b"=w24) -> ("y"=w493:dbl)
    "温度1" <- w493
    "波形图表" <- w493
    n302 = formula code="y=(x-a)/b;"("x"=w665, "a"=w21, "b"=w22) -> ("y"=w492:dbl)
    "温度2" <- w492
    "波形图表 4" <- w492
    n303 = formula code="y=(x-a)/b;"("x"=w661, "a"=w19, "b"=w20) -> ("y"=w491:dbl)
    "温度3" <- w491
    "波形图表 6" <- w491
    n304 = formula code="y=(x-a)/b;"("x"=w657, "a"=w17, "b"=w18) -> ("y"=w490:dbl)
    "温度4" <- w490
    "波形图表 8" <- w490
    n305 = formula code="y=(x-a)/b;"("x"=w653, "a"=w15, "b"=w16) -> ("y"=w458:dbl)
    "温度5" <- w458
    "波形图表 10" <- w458
    n306 = Index Array(array=w249, index=0 ("索引")) -> ()  [unwired: 1 out]
    n307 = Index Array(array=w249, index=1 ("索引")) -> ()  [unwired: 1 out]
    n308 = Index Array(array=w410, index=1 ("索引")) -> (element=w349:dbl)
    n309 = Index Array(array=w410, index=0 ("索引")) -> (element=w350:dbl)
    n310 = Index Array(array=w410, index=2 ("索引")) -> (element=w330:dbl)
    n311 = Index Array(array=w410, index=3 ("索引")) -> (element=w329:dbl)
    n312 = Index Array(array=w393, index=1 ("索引")) -> (element=w347:dbl)
    n313 = Index Array(array=w393, index=0 ("索引")) -> (element=w348:dbl)
    n314 = Index Array(array=w393, index=2 ("索引")) -> (element=w328:dbl)
    n315 = Index Array(array=w393, index=3 ("索引")) -> (element=w327:dbl)
    n316 = Index Array(array=w392, index=1 ("索引")) -> (element=w345:dbl)
    n317 = Index Array(array=w392, index=0 ("索引")) -> (element=w346:dbl)
    n318 = Index Array(array=w392, index=2 ("索引")) -> (element=w326:dbl)
    n319 = Index Array(array=w392, index=3 ("索引")) -> (element=w325:dbl)
    n320 = Index Array(array=w391, index=1 ("索引")) -> (element=w343:dbl)
    n321 = Index Array(array=w391, index=0 ("索引")) -> (element=w344:dbl)
    n322 = Index Array(array=w391, index=2 ("索引")) -> (element=w324:dbl)
    n323 = Index Array(array=w391, index=3 ("索引")) -> (element=w323:dbl)
    n324 = Index Array(array=w376, index=1 ("索引")) -> (element=w341:dbl)
    n325 = Index Array(array=w376, index=0 ("索引")) -> (element=w342:dbl)
    n326 = Index Array(array=w376, index=2 ("索引")) -> (element=w322:dbl)
    n327 = Index Array(array=w376, index=3 ("索引")) -> (element=w321:dbl)
    n328 = Index Array(array=w355, index=1 ("索引")) -> (element=w339:dbl)
    n329 = Index Array(array=w355, index=0 ("索引")) -> (element=w340:dbl)
    n330 = Index Array(array=w355, index=2 ("索引")) -> (element=w320:dbl)
    n331 = Index Array(array=w355, index=3 ("索引")) -> (element=w319:dbl)
    n332 = Index Array(array=w354, index=1 ("索引")) -> (element=w337:dbl)
    n333 = Index Array(array=w354, index=0 ("索引")) -> (element=w338:dbl)
    n334 = Index Array(array=w354, index=2 ("索引")) -> (element=w318:dbl)
    n335 = Index Array(array=w354, index=3 ("索引")) -> (element=w317:dbl)
    n336 = Index Array(array=w353, index=1 ("索引")) -> (element=w335:dbl)
    n337 = Index Array(array=w353, index=0 ("索引")) -> (element=w336:dbl)
    n338 = Index Array(array=w353, index=2 ("索引")) -> (element=w316:dbl)
    n339 = Index Array(array=w353, index=3 ("索引")) -> (element=w315:dbl)
    n340 = Index Array(array=w352, index=1 ("索引")) -> (element=w333:dbl)
    n341 = Index Array(array=w352, index=0 ("索引")) -> (element=w334:dbl)
    n342 = Index Array(array=w352, index=2 ("索引")) -> (element=w314:dbl)
    n343 = Index Array(array=w352, index=3 ("索引")) -> (element=w313:dbl)
    n344 = Index Array(array=w351, index=1 ("索引")) -> (element=w331:dbl)
    n345 = Index Array(array=w351, index=0 ("索引")) -> (element=w332:dbl)
    n346 = Index Array(array=w351, index=2 ("索引")) -> (element=w312:dbl)
    n347 = Index Array(array=w351, index=3 ("索引")) -> (element=w311:dbl)
    n348 = Index Array(array=w89, index=1 ("索引")) -> (element=w13:dbl)
    n349 = Index Array(array=w89, index=0 ("索引")) -> (element=w14:dbl)
    n350 = Index Array(array=w89, index=2 ("索引")) -> (element=w34:dbl)
    n351 = Index Array(array=w89, index=3 ("索引")) -> (element=w33:dbl)
    n352 = Index Array(array=w88, index=1 ("索引")) -> (element=w11:dbl)
    n353 = Index Array(array=w88, index=0 ("索引")) -> (element=w12:dbl)
    n354 = Index Array(array=w88, index=2 ("索引")) -> (element=w32:dbl)
    n355 = Index Array(array=w88, index=3 ("索引")) -> (element=w31:dbl)
    n356 = Index Array(array=w86, index=1 ("索引")) -> (element=w8:dbl)
    n357 = Index Array(array=w86, index=0 ("索引")) -> (element=w9:dbl)
    n358 = Index Array(array=w86, index=2 ("索引")) -> (element=w28:dbl)
    n359 = Index Array(array=w86, index=3 ("索引")) -> (element=w27:dbl)
    n360 = Index Array(array=w85, index=1 ("索引")) -> (element=w6:dbl)
    n361 = Index Array(array=w85, index=0 ("索引")) -> (element=w7:dbl)
    n362 = Index Array(array=w85, index=2 ("索引")) -> (element=w26:dbl)
    n363 = Index Array(array=w85, index=3 ("索引")) -> (element=w25:dbl)
    n364 = Index Array(array=w87, index=2 ("索引")) -> (element=w30:dbl)
    n365 = Index Array(array=w87, index=3 ("索引")) -> (element=w29:dbl)
    n366 = Index Array(array=w308, index=1 ("索引")) -> (element=w247:dbl)
    n367 = Index Array(array=w308, index=0 ("索引")) -> (element=w248:dbl)
    n368 = Index Array(array=w308, index=2 ("索引")) -> (element=w228:dbl)
    n369 = Index Array(array=w308, index=3 ("索引")) -> (element=w227:dbl)
    n370 = Index Array(array=w291, index=1 ("索引")) -> (element=w245:dbl)
    n371 = Index Array(array=w291, index=0 ("索引")) -> (element=w246:dbl)
    n372 = Index Array(array=w291, index=2 ("索引")) -> (element=w226:dbl)
    n373 = Index Array(array=w291, index=3 ("索引")) -> (element=w225:dbl)
    n374 = Index Array(array=w290, index=1 ("索引")) -> (element=w243:dbl)
    n375 = Index Array(array=w290, index=0 ("索引")) -> (element=w244:dbl)
    n376 = Index Array(array=w290, index=2 ("索引")) -> (element=w224:dbl)
    n377 = Index Array(array=w290, index=3 ("索引")) -> (element=w223:dbl)
    n378 = Index Array(array=w289, index=1 ("索引")) -> (element=w241:dbl)
    n379 = Index Array(array=w289, index=0 ("索引")) -> (element=w242:dbl)
    n380 = Index Array(array=w289, index=2 ("索引")) -> (element=w222:dbl)
    n381 = Index Array(array=w289, index=3 ("索引")) -> (element=w221:dbl)
    n382 = Index Array(array=w274, index=1 ("索引")) -> (element=w239:dbl)
    n383 = Index Array(array=w274, index=0 ("索引")) -> (element=w240:dbl)
    n384 = Index Array(array=w274, index=2 ("索引")) -> (element=w220:dbl)
    n385 = Index Array(array=w274, index=3 ("索引")) -> (element=w219:dbl)
    n386 = Index Array(array=w253, index=1 ("索引")) -> (element=w237:dbl)
    n387 = Index Array(array=w253, index=0 ("索引")) -> (element=w238:dbl)
    n388 = Index Array(array=w253, index=2 ("索引")) -> (element=w218:dbl)
    n389 = Index Array(array=w253, index=3 ("索引")) -> (element=w217:dbl)
    n390 = Index Array(array=w252, index=1 ("索引")) -> (element=w235:dbl)
    n391 = Index Array(array=w252, index=0 ("索引")) -> (element=w236:dbl)
    n392 = Index Array(array=w252, index=2 ("索引")) -> (element=w216:dbl)
    n393 = Index Array(array=w252, index=3 ("索引")) -> (element=w215:dbl)
    n394 = Index Array(array=w251, index=1 ("索引")) -> (element=w233:dbl)
    n395 = Index Array(array=w251, index=0 ("索引")) -> (element=w234:dbl)
    n396 = Index Array(array=w251, index=2 ("索引")) -> (element=w214:dbl)
    n397 = Index Array(array=w251, index=3 ("索引")) -> (element=w213:dbl)
    n398 = Index Array(array=w250, index=1 ("索引")) -> (element=w231:dbl)
    n399 = Index Array(array=w250, index=0 ("索引")) -> (element=w232:dbl)
    n400 = Index Array(array=w250, index=2 ("索引")) -> (element=w212:dbl)
    n401 = Index Array(array=w250, index=3 ("索引")) -> (element=w211:dbl)
    n402 = Index Array(array=w206, index=1 ("索引")) -> (element=w83:dbl)
    n403 = Index Array(array=w206, index=0 ("索引")) -> (element=w84:dbl)
    n404 = Index Array(array=w206, index=2 ("索引")) -> (element=w64:dbl)
    n405 = Index Array(array=w206, index=3 ("索引")) -> (element=w63:dbl)
    n406 = Index Array(array=w189, index=1 ("索引")) -> (element=w81:dbl)
    n407 = Index Array(array=w189, index=0 ("索引")) -> (element=w82:dbl)
    n408 = Index Array(array=w189, index=2 ("索引")) -> (element=w62:dbl)
    n409 = Index Array(array=w189, index=3 ("索引")) -> (element=w61:dbl)
    n410 = Index Array(array=w188, index=1 ("索引")) -> (element=w79:dbl)
    n411 = Index Array(array=w188, index=0 ("索引")) -> (element=w80:dbl)
    n412 = Index Array(array=w188, index=2 ("索引")) -> (element=w60:dbl)
    n413 = Index Array(array=w188, index=3 ("索引")) -> (element=w59:dbl)
    n414 = Index Array(array=w187, index=1 ("索引")) -> (element=w77:dbl)
    n415 = Index Array(array=w187, index=0 ("索引")) -> (element=w78:dbl)
    n416 = Index Array(array=w187, index=2 ("索引")) -> (element=w58:dbl)
    n417 = Index Array(array=w187, index=3 ("索引")) -> (element=w57:dbl)
    n418 = Index Array(array=w172, index=1 ("索引")) -> (element=w75:dbl)
    n419 = Index Array(array=w172, index=0 ("索引")) -> (element=w76:dbl)
    n420 = Index Array(array=w172, index=2 ("索引")) -> (element=w56:dbl)
    n421 = Index Array(array=w172, index=3 ("索引")) -> (element=w55:dbl)
    n422 = Index Array(array=w151, index=1 ("索引")) -> (element=w73:dbl)
    n423 = Index Array(array=w151, index=0 ("索引")) -> (element=w74:dbl)
    n424 = Index Array(array=w151, index=2 ("索引")) -> (element=w54:dbl)
    n425 = Index Array(array=w151, index=3 ("索引")) -> (element=w53:dbl)
    n426 = Index Array(array=w150, index=1 ("索引")) -> (element=w71:dbl)
    n427 = Index Array(array=w150, index=0 ("索引")) -> (element=w72:dbl)
    n428 = Index Array(array=w150, index=2 ("索引")) -> (element=w52:dbl)
    n429 = Index Array(array=w150, index=3 ("索引")) -> (element=w51:dbl)
    n430 = Index Array(array=w149, index=1 ("索引")) -> (element=w69:dbl)
    n431 = Index Array(array=w149, index=0 ("索引")) -> (element=w70:dbl)
    n432 = Index Array(array=w149, index=2 ("索引")) -> (element=w50:dbl)
    n433 = Index Array(array=w149, index=3 ("索引")) -> (element=w49:dbl)
    n434 = Index Array(array=w148, index=0 ("索引")) -> (element=w65:dbl)
    n435 = Index Array(array=w148, index=1 ("索引")) -> (element=w66:dbl)
    n436 = Index Array(array=w148, index=2 ("索引")) -> (element=w48:dbl)
    n437 = Index Array(array=w148, index=3 ("索引")) -> (element=w47:dbl)
    n438 = Index Array(array=w147, index=1 ("索引")) -> (element=w67:dbl)
    n439 = Index Array(array=w147, index=0 ("索引")) -> (element=w68:dbl)
    n440 = Index Array(array=w147, index=2 ("索引")) -> (element=w46:dbl)
    n441 = Index Array(array=w147, index=3 ("索引")) -> (element=w45:dbl)
    n442 = Index Array(array=w87, index=0 ("索引")) -> (element=w10:dbl)
    n443 = Format Date/Time String() -> (date/time string=w708:string)  [unwired: 3 in]
    n444 = formula code="y=(x-a)/b;"("x"=w631, "a"=w349, "b"=w350) -> ("y"=w489:dbl)
    "温度1 2" <- w489
    "波形图表 22" <- w489
    n445 = formula code="y=(x-a)/b;"("x"=w627, "a"=w347, "b"=w348) -> ("y"=w488:dbl)
    "温度2 2" <- w488
    "波形图表 24" <- w488
    n446 = formula code="y=(x-a)/b;"("x"=w623, "a"=w345, "b"=w346) -> ("y"=w487:dbl)
    "温度3 2" <- w487
    "波形图表 26" <- w487
    n447 = formula code="y=(x-a)/b;"("x"=w619, "a"=w343, "b"=w344) -> ("y"=w486:dbl)
    "温度4 2" <- w486
    "波形图表 28" <- w486
    n448 = formula code="y=(x-a)/b;"("x"=w615, "a"=w341, "b"=w342) -> ("y"=w485:dbl)
    "温度5 2" <- w485
    "波形图表 30" <- w485
    n449 = formula code="y=(x-a)/b;"("x"=w611, "a"=w339, "b"=w340) -> ("y"=w484:dbl)
    "温度6 2" <- w484
    "波形图表 32" <- w484
    n450 = formula code="y=(x-a)/b;"("x"=w607, "a"=w337, "b"=w338) -> ("y"=w483:dbl)
    "温度7 2" <- w483
    "波形图表 34" <- w483
    n451 = formula code="y=(x-a)/b;"("x"=w603, "a"=w335, "b"=w336) -> ("y"=w482:dbl)
    "温度8 2" <- w482
    "波形图表 36" <- w482
    n452 = formula code="y=(x-a)/b;"("x"=w599, "a"=w333, "b"=w334) -> ("y"=w481:dbl)
    "温度9 2" <- w481
    "波形图表 38" <- w481
    n453 = formula code="y=(x-a)/b;"("x"=w595, "a"=w331, "b"=w332) -> ("y"=w480:dbl)
    "温度10 2" <- w480
    "波形图表 40" <- w480
    n454 = formula code="y=(x-a)/b;"("x"=w649, "a"=w13, "b"=w14) -> ("y"=w457:dbl)
    "温度6" <- w457
    "波形图表 12" <- w457
    n455 = formula code="y=(x-a)/b;"("x"=w643, "a"=w10, "b"=w10) -> ("y"=w455:dbl)
    "温度8" <- w455
    "波形图表 16" <- w455
    n456 = formula code="y=(x-a)/b;"("x"=w639, "a"=w8, "b"=w9) -> ("y"=w454:dbl)
    "温度9" <- w454
    "波形图表 18" <- w454
    n457 = formula code="y=(x-a)/b;"("x"=w635, "a"=w6, "b"=w7) -> ("y"=w453:dbl)
    "温度10" <- w453
    "波形图表 20" <- w453
    n458 = formula code="y=(x-a)/b;"("x"=w229, "a"=w11, "b"=w12) -> ("y"=w456:dbl)
    "温度7" <- w456
    "波形图表 14" <- w456
    n459 = formula code="y=(x-a)/b;"("x"=w516, "a"=w229, "b"=w230) -> ("y"=w459:dbl)
    "温度10 4" <- w459
    "波形图表 80" <- w459
    n460 = formula code="y=(x-a)/b;"("x"=w552, "a"=w247, "b"=w248) -> ("y"=w468:dbl)
    "温度1 4" <- w468
    "波形图表 62" <- w468
    n461 = formula code="y=(x-a)/b;"("x"=w548, "a"=w245, "b"=w246) -> ("y"=w467:dbl)
    "温度2 4" <- w467
    "波形图表 72" <- w467
    n462 = formula code="y=(x-a)/b;"("x"=w544, "a"=w243, "b"=w244) -> ("y"=w466:dbl)
    "温度3 4" <- w466
    "波形图表 64" <- w466
    n463 = formula code="y=(x-a)/b;"("x"=w540, "a"=w241, "b"=w242) -> ("y"=w465:dbl)
    "温度4 4" <- w465
    "波形图表 74" <- w465
    n464 = formula code="y=(x-a)/b;"("x"=w536, "a"=w239, "b"=w240) -> ("y"=w464:dbl)
    "温度5 4" <- w464
    "波形图表 66" <- w464
    n465 = formula code="y=(x-a)/b;"("x"=w532, "a"=w237, "b"=w238) -> ("y"=w463:dbl)
    "温度6 4" <- w463
    "波形图表 76" <- w463
    n466 = formula code="y=(x-a)/b;"("x"=w528, "a"=w235, "b"=w236) -> ("y"=w462:dbl)
    "温度7 4" <- w462
    "波形图表 68" <- w462
    n467 = formula code="y=(x-a)/b;"("x"=w524, "a"=w233, "b"=w234) -> ("y"=w461:dbl)
    "温度8 4" <- w461
    "波形图表 78" <- w461
    n468 = formula code="y=(x-a)/b;"("x"=w520, "a"=w231, "b"=w232) -> ("y"=w460:dbl)
    "温度9 4" <- w460
    "波形图表 70" <- w460
    n469 = formula code="y=(x-a)/b;"("x"=w591, "a"=w83, "b"=w84) -> ("y"=w479:dbl)
    "温度1 3" <- w479
    "波形图表 42" <- w479
    n470 = formula code="y=(x-a)/b;"("x"=w587, "a"=w81, "b"=w82) -> ("y"=w478:dbl)
    "温度2 3" <- w478
    "波形图表 44" <- w478
    n471 = formula code="y=(x-a)/b;"("x"=w583, "a"=w79, "b"=w80) -> ("y"=w477:dbl)
    "温度3 3" <- w477
    "波形图表 46" <- w477
    n472 = formula code="y=(x-a)/b;"("x"=w579, "a"=w77, "b"=w78) -> ("y"=w476:dbl)
    "温度4 3" <- w476
    "波形图表 48" <- w476
    n473 = formula code="y=(x-a)/b;"("x"=w575, "a"=w75, "b"=w76) -> ("y"=w475:dbl)
    "温度5 3" <- w475
    "波形图表 50" <- w475
    n474 = formula code="y=(x-a)/b;"("x"=w474, "a"=w73, "b"=w74) -> ("y"=w473:dbl)
    "温度6 3" <- w473
    "波形图表 52" <- w473
    n475 = formula code="y=(x-a)/b;"("x"=w568, "a"=w71, "b"=w72) -> ("y"=w472:dbl)
    "温度7 3" <- w472
    "波形图表 54" <- w472
    n476 = formula code="y=(x-a)/b;"("x"=w564, "a"=w69, "b"=w70) -> ("y"=w471:dbl)
    "温度8 3" <- w471
    "波形图表 56" <- w471
    n477 = formula code="y=(x-a)/b;"("x"=w560, "a"=w65, "b"=w66) -> ("y"=w470:dbl)
    "温度9 3" <- w470
    "波形图表 58" <- w470
    n478 = formula code="y=(x-a)/b;"("x"=w556, "a"=w67, "b"=w68) -> ("y"=w469:dbl)
    "温度10 3" <- w469
    "波形图表 60" <- w469
    n479 = Index Array(array=w249, index=2 ("索引")) -> (element=w210:dbl)
    n480 = Index Array(array=w249, index=3 ("索引")) -> (element=w209:dbl)
    n481 = Scan From String(format string="%d/%d/%d %d:%d:%d" ("格式字符串"), input string=w708) -> (output 1=w719:i32, output 2=w717:i32, output 3=w709:i32, output 4=w710:i32, output 5=w711:i32, output 6=w704:i32)  [unwired: 8 in, 3 out]
    n482 = formula code="y=(x-0.01*t-a)/k;"("x"=w667, "a"=w43, "k"=w44, "t"=w493) -> ("y"=w432:dbl)
    "湿度1" <- w432
    "波形图表 2" <- w432
    n483 = formula code="y=(x-0.01*t-a)/k;"("x"=w663, "a"=w41, "k"=w42, "t"=w492) -> ("y"=w431:dbl)
    "湿度2" <- w431
    "波形图表 3" <- w431
    n484 = formula code="y=(x-0.01*t-a)/k;"("x"=w659, "a"=w39, "k"=w40, "t"=w491) -> ("y"=w430:dbl)
    "湿度3" <- w430
    "波形图表 5" <- w430
    n485 = formula code="y=(x-0.01*t-a)/k;"("x"=w655, "a"=w37, "k"=w38, "t"=w490) -> ("y"=w429:dbl)
    "湿度4" <- w429
    "波形图表 7" <- w429
    n486 = formula code="y=(x-0.01*t-a)/k;"("x"=w651, "a"=w35, "k"=w36, "t"=w458) -> ("y"=w428:dbl)
    "湿度5" <- w428
    "波形图表 9" <- w428
    n487 = Format Into String(format string="%d" ("格式字符串"), w719) -> (resulting string=w714:string)  [unwired: 2 in, 1 out]
    n488 = Format Into String(format string="%d" ("格式字符串"), w717) -> (resulting string=w713:string)  [unwired: 2 in, 1 out]
    n489 = Format Into String(format string="%d" ("格式字符串"), w709) -> (resulting string=w712:string)  [unwired: 2 in, 1 out]
    n490 = Multiply(x=w711, y=100) -> (x*y=w706:i32)
    n491 = formula code="y=(x-0.01*t-a)/k;"("x"=w629, "a"=w329, "k"=w330, "t"=w489) -> ("y"=w452:dbl)
    "湿度1 2" <- w452
    "波形图表 21" <- w452
    n492 = formula code="y=(x-0.01*t-a)/k;"("x"=w625, "a"=w327, "k"=w328, "t"=w488) -> ("y"=w451:dbl)
    "湿度2 2" <- w451
    "波形图表 23" <- w451
    n493 = formula code="y=(x-0.01*t-a)/k;"("x"=w621, "a"=w325, "k"=w326, "t"=w487) -> ("y"=w450:dbl)
    "湿度3 2" <- w450
    "波形图表 25" <- w450
    n494 = formula code="y=(x-0.01*t-a)/k;"("x"=w617, "a"=w323, "k"=w324, "t"=w486) -> ("y"=w449:dbl)
    "湿度4 2" <- w449
    "波形图表 27" <- w449
    n495 = formula code="y=(x-0.01*t-a)/k;"("x"=w613, "a"=w321, "k"=w322, "t"=w485) -> ("y"=w448:dbl)
    "湿度5 2" <- w448
    "波形图表 29" <- w448
    n496 = formula code="y=(x-0.01*t-a)/k;"("x"=w609, "a"=w319, "k"=w320, "t"=w484) -> ("y"=w447:dbl)
    "湿度6 2" <- w447
    "波形图表 31" <- w447
    n497 = formula code="y=(x-0.01*t-a)/k;"("x"=w605, "a"=w317, "k"=w318, "t"=w483) -> ("y"=w446:dbl)
    "湿度7 2" <- w446
    "波形图表 33" <- w446
    n498 = formula code="y=(x-0.01*t-a)/k;"("x"=w601, "a"=w315, "k"=w316, "t"=w482) -> ("y"=w445:dbl)
    "湿度8 2" <- w445
    "波形图表 35" <- w445
    n499 = formula code="y=(x-0.01*t-a)/k;"("x"=w597, "a"=w313, "k"=w314, "t"=w481) -> ("y"=w444:dbl)
    "湿度9 2" <- w444
    "波形图表 37" <- w444
    n500 = formula code="y=(x-0.01*t-a)/k;"("x"=w593, "a"=w311, "k"=w312, "t"=w480) -> ("y"=w443:dbl)
    "湿度10 2" <- w443
    "波形图表 39" <- w443
    n501 = formula code="y=(x-0.01*t-a)/k;"("x"=w641, "a"=w29, "k"=w30, "t"=w455) -> ("y"=w425:dbl)
    "湿度8" <- w425
    "波形图表 15" <- w425
    n502 = formula code="y=(x-0.01*t-a)/k;"("x"=w230, "a"=w33, "k"=w34, "t"=w457) -> ("y"=w427:dbl)
    "湿度6" <- w427
    "波形图表 11" <- w427
    n503 = formula code="y=(x-0.01*t-a)/k;"("x"=w637, "a"=w27, "k"=w28, "t"=w454) -> ("y"=w424:dbl)
    "湿度9" <- w424
    "波形图表 17" <- w424
    n504 = formula code="y=(x-0.01*t-a)/k;"("x"=w645, "a"=w31, "k"=w32, "t"=w456) -> ("y"=w426:dbl)
    "湿度7" <- w426
    "波形图表 13" <- w426
    n505 = formula code="y=(x-0.01*t-a)/k;"("x"=w633, "a"=w25, "k"=w26, "t"=w453) -> ("y"=w423:dbl)
    "湿度10" <- w423
    "波形图表 19" <- w423
    n506 = formula code="y=(x-0.01*t-a)/k;"("x"=w550, "a"=w227, "k"=w228, "t"=w468) -> ("y"=w422:dbl)
    "湿度1 4" <- w422
    "波形图表 61" <- w422
    n507 = formula code="y=(x-0.01*t-a)/k;"("x"=w546, "a"=w225, "k"=w226, "t"=w467) -> ("y"=w421:dbl)
    "湿度2 4" <- w421
    "波形图表 71" <- w421
    n508 = formula code="y=(x-0.01*t-a)/k;"("x"=w542, "a"=w223, "k"=w224, "t"=w466) -> ("y"=w420:dbl)
    "湿度3 4" <- w420
    "波形图表 63" <- w420
    n509 = formula code="y=(x-0.01*t-a)/k;"("x"=w538, "a"=w221, "k"=w222, "t"=w465) -> ("y"=w419:dbl)
    "湿度4 4" <- w419
    "波形图表 73" <- w419
    n510 = formula code="y=(x-0.01*t-a)/k;"("x"=w514, "a"=w209, "k"=w210, "t"=w459) -> ("y"=w413:dbl)
    "湿度10 4" <- w413
    "波形图表 79" <- w413
    n511 = formula code="y=(x-0.01*t-a)/k;"("x"=w534, "a"=w219, "k"=w220, "t"=w464) -> ("y"=w418:dbl)
    "湿度5 4" <- w418
    "波形图表 65" <- w418
    n512 = formula code="y=(x-0.01*t-a)/k;"("x"=w530, "a"=w217, "k"=w218, "t"=w463) -> ("y"=w417:dbl)
    "湿度6 4" <- w417
    "波形图表 75" <- w417
    n513 = formula code="y=(x-0.01*t-a)/k;"("x"=w526, "a"=w215, "k"=w216, "t"=w462) -> ("y"=w416:dbl)
    "湿度7 4" <- w416
    "波形图表 67" <- w416
    n514 = formula code="y=(x-0.01*t-a)/k;"("x"=w522, "a"=w213, "k"=w214, "t"=w461) -> ("y"=w415:dbl)
    "湿度8 4" <- w415
    "波形图表 77" <- w415
    n515 = formula code="y=(x-0.01*t-a)/k;"("x"=w518, "a"=w211, "k"=w212, "t"=w460) -> ("y"=w414:dbl)
    "湿度9 4" <- w414
    "波形图表 69" <- w414
    n516 = formula code="y=(x-0.01*t-a)/k;"("x"=w589, "a"=w63, "k"=w64, "t"=w479) -> ("y"=w442:dbl)
    "湿度1 3" <- w442
    "波形图表 41" <- w442
    n517 = formula code="y=(x-0.01*t-a)/k;"("x"=w585, "a"=w61, "k"=w62, "t"=w478) -> ("y"=w441:dbl)
    "湿度2 3" <- w441
    "波形图表 43" <- w441
    n518 = formula code="y=(x-0.01*t-a)/k;"("x"=w581, "a"=w59, "k"=w60, "t"=w477) -> ("y"=w440:dbl)
    "湿度3 3" <- w440
    "波形图表 45" <- w440
    n519 = formula code="y=(x-0.01*t-a)/k;"("x"=w577, "a"=w57, "k"=w58, "t"=w476) -> ("y"=w439:dbl)
    "湿度4 3" <- w439
    "波形图表 47" <- w439
    n520 = formula code="y=(x-0.01*t-a)/k;"("x"=w573, "a"=w55, "k"=w56, "t"=w475) -> ("y"=w438:dbl)
    "湿度5 3" <- w438
    "波形图表 49" <- w438
    n521 = formula code="y=(x-0.01*t-a)/k;"("x"=w570, "a"=w53, "k"=w54, "t"=w473) -> ("y"=w437:dbl)
    "湿度6 3" <- w437
    "波形图表 51" <- w437
    n522 = formula code="y=(x-0.01*t-a)/k;"("x"=w566, "a"=w51, "k"=w52, "t"=w472) -> ("y"=w436:dbl)
    "湿度7 3" <- w436
    "波形图表 53" <- w436
    n523 = formula code="y=(x-0.01*t-a)/k;"("x"=w562, "a"=w49, "k"=w50, "t"=w471) -> ("y"=w435:dbl)
    "湿度8 3" <- w435
    "波形图表 55" <- w435
    n524 = formula code="y=(x-0.01*t-a)/k;"("x"=w558, "a"=w47, "k"=w48, "t"=w470) -> ("y"=w434:dbl)
    "湿度9 3" <- w434
    "波形图表 57" <- w434
    n525 = formula code="y=(x-0.01*t-a)/k;"("x"=w554, "a"=w45, "k"=w46, "t"=w469) -> ("y"=w433:dbl)
    "湿度10 3" <- w433
    "波形图表 59" <- w433
    n526 = Multiply(x=w710, y=10000) -> (x*y=w707:i32)
    n527 = Add(x=w707, y=w706) -> (x+y=w705:i32)
    n528 = Build Array(w493, w432, w492, w431, w491, w430) -> (w512:dbl[])
    n529 = Concatenate Strings(w714, w713, w712) -> (w677:string)
    n530 = Build Array(w489, w452, w488, w451, w487, w450) -> (w508:dbl[])
    n531 = Build Array(w486, w449, w485, w448, w484, w447) -> (w507:dbl[])
    n532 = Build Array(w483, w446, w482, w445, w481, w444, w480, w443) -> (w506:dbl[])
    n533 = Build Array(w490, w429, w458, w428, w457, w427) -> (w511:dbl[])
    n534 = Build Array(w456, w426, w455, w425, w454, w424, w453, w423) -> (w510:dbl[])
    n535 = Build Array(w468, w422, w467, w421, w466, w420) -> (w496:dbl[])
    n536 = Build Array(w465, w419, w464, w418, w463, w417) -> (w495:dbl[])
    n537 = Build Array(w462, w416, w461, w415, w460, w414, w459, w413) -> (w498:dbl[])
    n538 = Build Array(w479, w442, w478, w441, w477, w440) -> (w502:dbl[])
    n539 = Build Array(w476, w439, w475, w438, w473, w437) -> (w501:dbl[])
    n540 = Build Array(w472, w436, w471, w435, w470, w434, w469, w433) -> (w500:dbl[])
    n541 = Concatenate Strings(w677, "通道" ("字符串"), "2" ("字符串")) -> (w694:string)
    n542 = Concatenate Strings(w677, "通道" ("字符串"), "1" ("字符串")) -> (w700:string)
    n543 = Concatenate Strings(w677, "通道" ("字符串"), "4" ("字符串")) -> (w682:string)
    n544 = Concatenate Strings(w677, "通道" ("字符串"), "3" ("字符串")) -> (w688:string)
    n545 = Build Array (concatenate)(w505, w508, w507, w506) -> (w504:dbl[])
    n546 = Build Array (concatenate)(w513, w512, w511, w510) -> (w509:dbl[])
    n547 = Build Array (concatenate)(w497, w496, w495, w498) -> (w494:dbl[])
    n548 = Build Array (concatenate)(w503, w502, w501, w500) -> (w499:dbl[])
    n549 = Add(x=w705, y=w704) -> (x+y=w679:i32)
    n550 = Build Array (concatenate)(w679, w504) -> (w697:dbl[])
    n551 = Build Array (concatenate)(w679, w509) -> (w703:dbl[])
    n552 = Build Array (concatenate)(w679, w494) -> (w685:dbl[])
    n553 = Build Array (concatenate)(w679, w499) -> (w691:dbl[])
    n554 = Build Path(base path=w678, name or relative path=w694) -> (appended path=w696:path)
    n555 = Build Path(base path=w678, name or relative path=w700) -> (appended path=w702:path)
    n556 = Build Path(base path=w678, name or relative path=w682) -> (appended path=w684:path)
    n557 = Build Path(base path=w678, name or relative path=w688) -> (appended path=w690:path)
    n558 = call-poly <vilib>:"Write To Spreadsheet File.vi"("append to file? (new file:F)"=TRUE, "1D data"=w697, "file path (dialog if empty)"=w696) -> ()  [unwired: 5 in, 1 out]
    n559 = call-poly <vilib>:"Write To Spreadsheet File.vi"("append to file? (new file:F)"=TRUE, "1D data"=w703, "file path (dialog if empty)"=w702) -> ()  [unwired: 5 in, 1 out]
    n560 = call-poly <vilib>:"Write To Spreadsheet File.vi"("append to file? (new file:F)"=TRUE, "1D data"=w685, "file path (dialog if empty)"=w684) -> ()  [unwired: 5 in, 1 out]
    n561 = call-poly <vilib>:"Write To Spreadsheet File.vi"("append to file? (new file:F)"=TRUE, "1D data"=w691, "file path (dialog if empty)"=w690) -> ()  [unwired: 5 in, 1 out]
  }
  n562 = VISA Close(VISA resource name=w2, error in (no error)=w1) -> (error out=w3:errorcluster)
  n563 = call <vilib>:"Clear Errors.vi"("error in (no error)"=w3) -> ()  [unwired: 5 in, 2 out]
